vi "PromptToRecord.vi"(8 "error in (no error)":errorcluster) -> (0 "error out":errorcluster, 2 "Record?":bool)   [LabVIEW 2011, in "UI_Interaction_Manager.lvclass"]
uses:
  UI_Interaction_Manager.lvclass
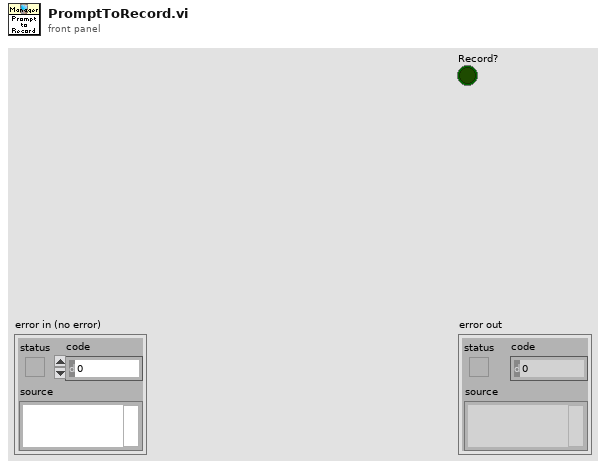
[diagram p1: front panel]
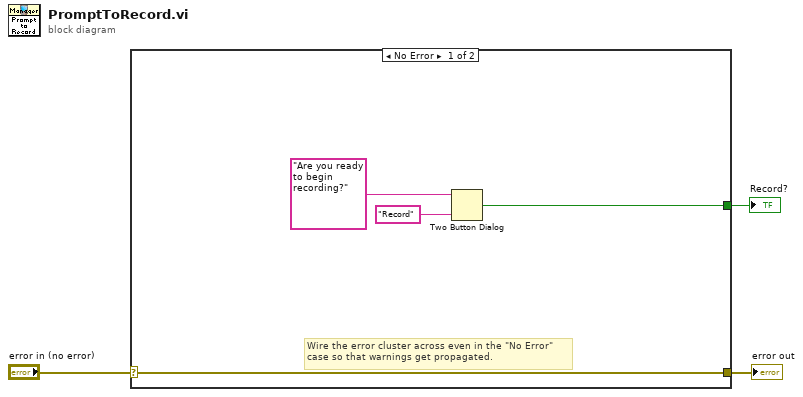
[diagram p0: block diagram]
diagram:
  n1 = case shown="No Error" "error in (no error)" {
    selector: "error in (no error)" -> [w7 w8]
    tunnel: [w7 w8] -> w2
    tunnel: [w4 _] -> w1
    frame No Error {
      # "Wire the error cluster across even in the \"No Error\"\ncase so that warnings get propagated."
      n2 = Two Button Dialog(message="Are you ready to begin recording?", 2:"Record" ("T button name (\"OK\")")) -> (T button?=w4:bool)  [unwired: 1 in]
    }
    frame Error {
    }
  }
  "error out" <- w2
  "Record?" <- w1
